vi "antonio-alexander Build.vi"(8 "error in (no error)":errorcluster) -> (0 "error out":errorcluster)   [LabVIEW 2015, in "lv-build-interface.lvlib"]
doc: "Build can be used to load a lv-builder class and build/post/deploy one or more build distributions for a loaded project."
uses:
  lv-build-interface.lvlib
  private/_controls/hmi_references.ctl
  private/_controls/hmi_states.ctl
  private/_controls/event_common.ctl
  private/_controls/event_common_command.ctl
  lv-build/public/_controls/configuration_command.ctl
  lv-builder/lv-builder.lvclass
  lv-build/lv-build.lvlib
panel:
  in  "update_version":bool
  in  "set_version":bool
  in  "select_project":bool
  in  "dependencies":bool
  in  "open_dist_folder":bool
  in  "load_class":bool
  in  "configure":bool
  in  "build":bool
  in  "post":bool
  in  "start":bool
  in  "cancel":bool
  in  "deploy":bool
  in  "exit":bool
  out "builder_class":string caption="Builder Class"
  in  "targets_artifacts_tree":string[](tree)=["0"]
  out "version":string caption="Version"
  out "git_commit_hash":string caption="Git Commit Hash"
  out "progress_bar":dbl(slide) caption="Progress" scale=0.0..100.0
  out "status":string caption="Status"
  out "project_file":string caption="Project"
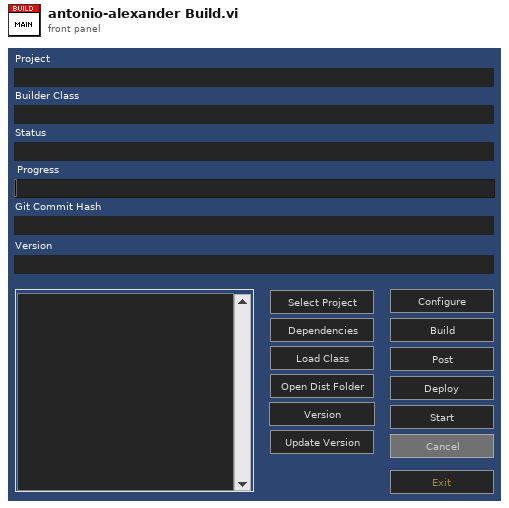
[diagram p1: front panel]
types:
  T1 = typedef "lv-build-interface.lvlib/event_common.ctl" = cluster{"command":T2, "data":variant}
  T2 = typedef "lv-build-interface.lvlib/event_common_command.ctl" = enum16{"<command>", "die", "<null>"}
  T3 = typedef "lv-build-interface.lvlib/hmi_references.ctl" = cluster{"vi_reference":refnum<vi>, "status":refnum<vi>, "progress":refnum<vi>, "tree":refnum<vi>, "project_file":refnum<vi>, "commit_hash":refnum<vi>, "version":refnum<vi>, "build":refnum<vi>, "cancel":refnum<vi>, "post":refnum<vi>, "start":refnum<vi>, "builder_class":refnum<vi>, "deploy":refnum<vi>}
  T4 = typedef "lv-build-interface.lvlib/hmi_states.ctl" = enum16{"<hmi_states>", "initialize", "check_ui", "shutdown", "<null>"}
  T5 = typedef "lv-build.lvlib/configuration_command.ctl" = enum16{"<config_command>", "read_config", "write_config", "<null>"}
  T6 = typedef "lv-build-interface.lvlib/action.ctl" = enum16{"<action>", "build", "post", "deploy", "<null>"}
  T7 = typedef "lv-build.lvlib/build_specification.ctl" = cluster{"type":T8, "build_spec_name":string, "target_name":string, "owner_name []":string[], "project_path":path, "build_destination":path, "build_artifact":path, "post_artifact":path}
  T8 = typedef "lv-build.lvlib/build_type.ctl" = enum16{"<build_type>", "application_pc", "application_rt", "installer", "llb", "lvlibp", "zip", "fpga", "<null>"}
  T9 = typedef "lv-build.lvlib/configuration.ctl" = cluster{"project_file":string, "build_class_file":string}
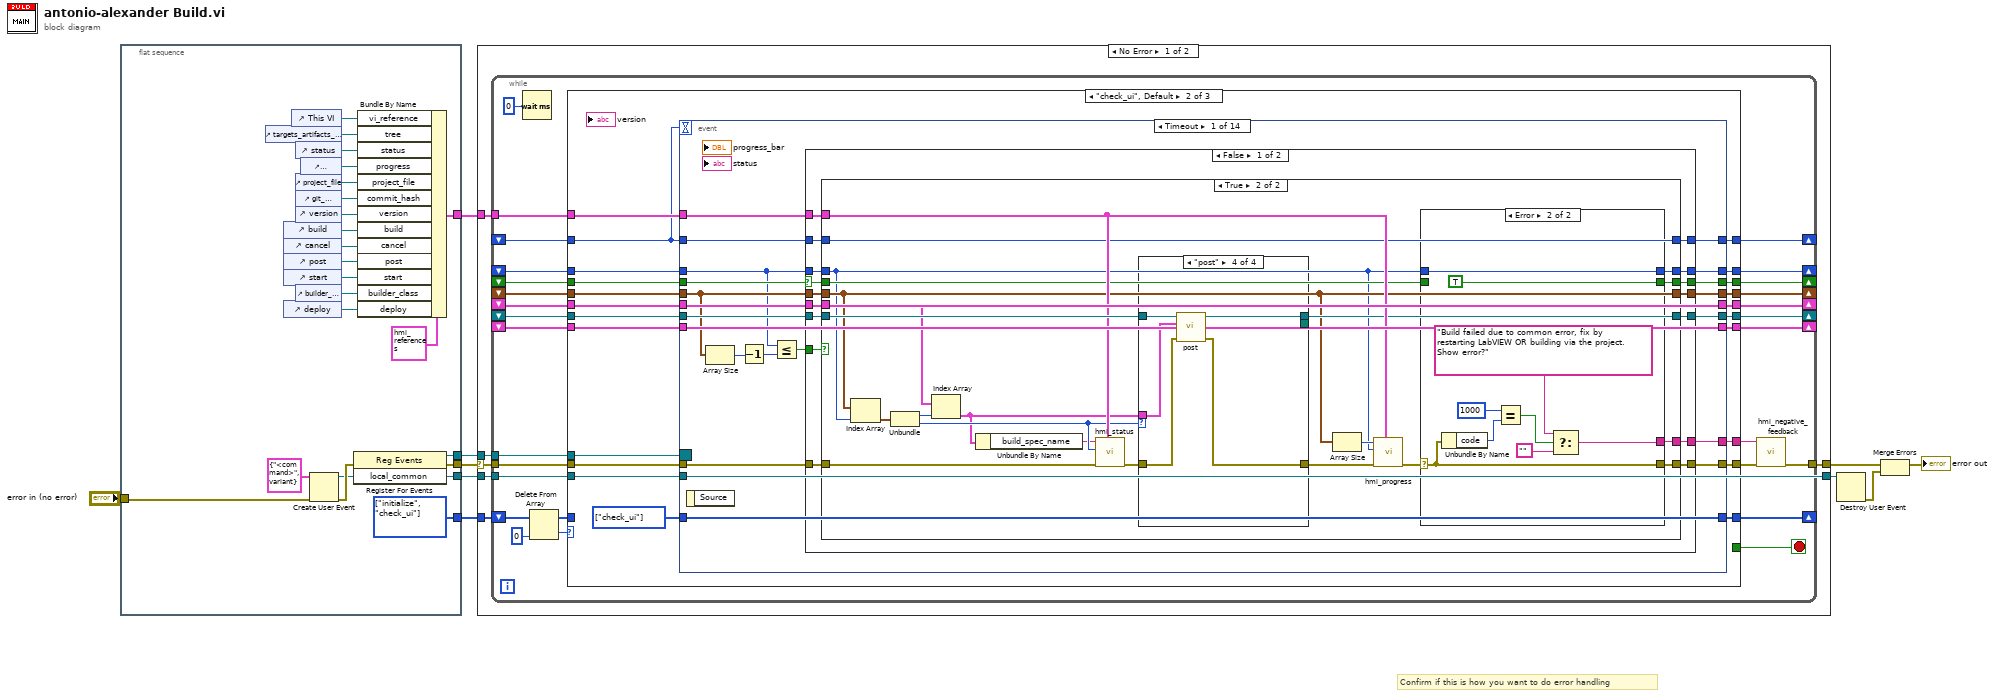
[diagram p0: block diagram]
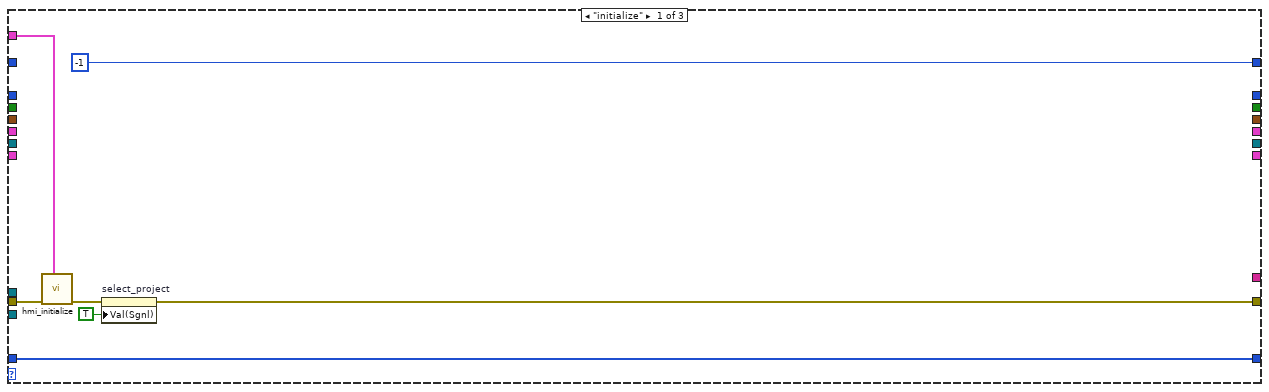
[diagram p2: hidden frame]
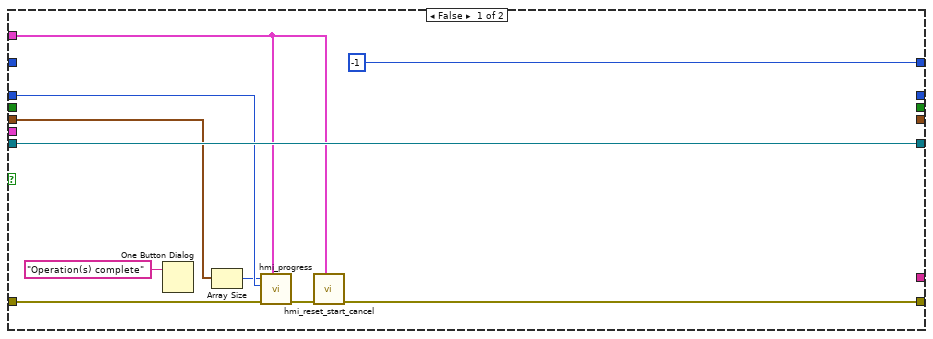
[diagram p3: hidden frame]
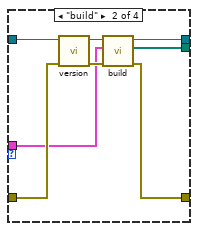
[diagram p5: hidden frame]
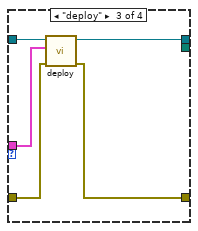
[diagram p6: hidden frame]
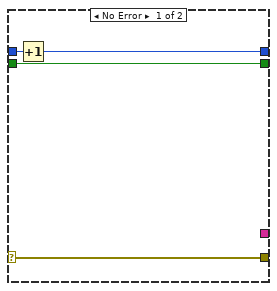
[diagram p7: hidden frame]
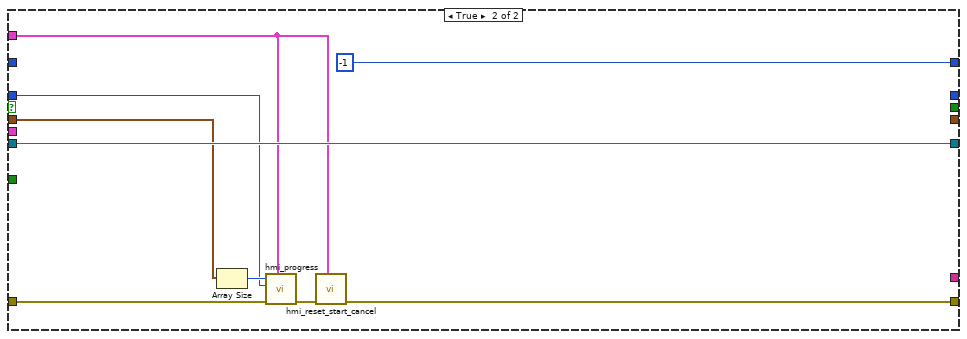
[diagram p8: hidden frame]
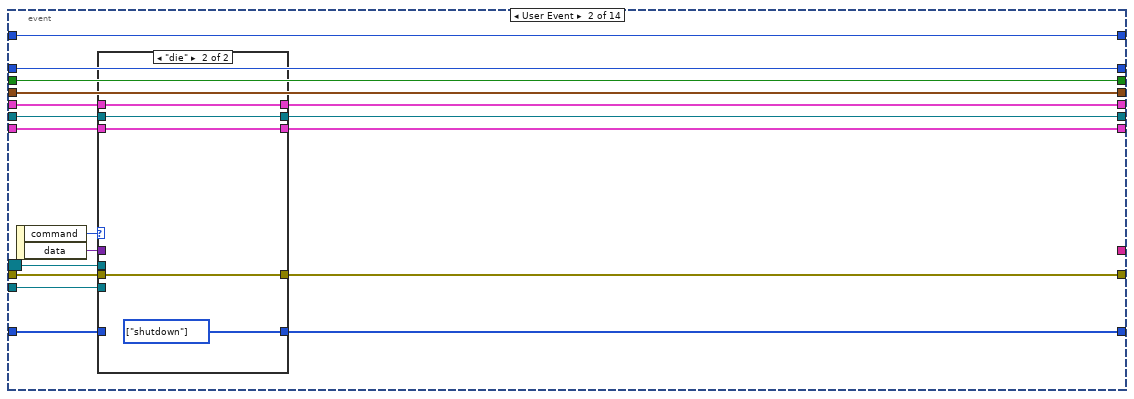
[diagram p9: hidden frame]
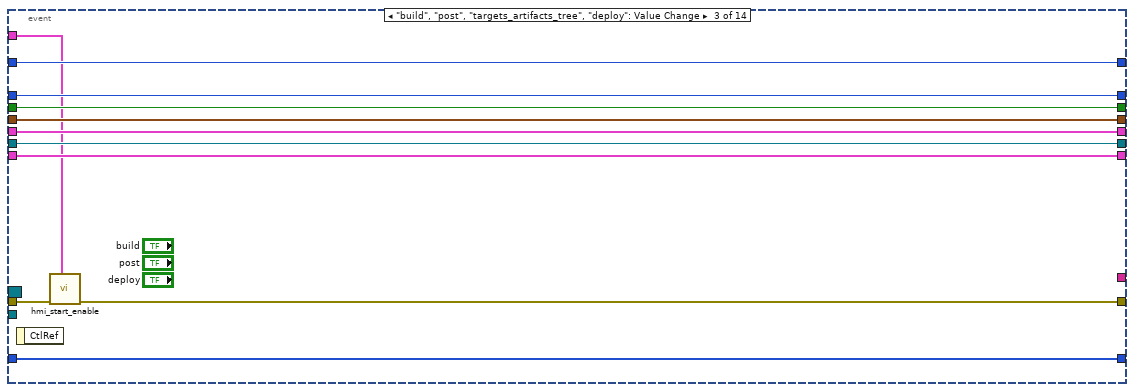
[diagram p11: hidden frame]
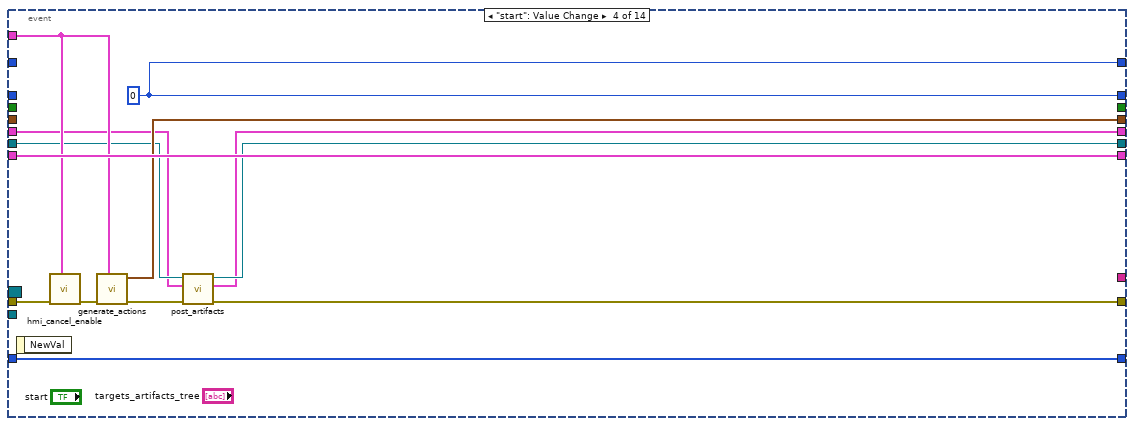
[diagram p12: hidden frame]
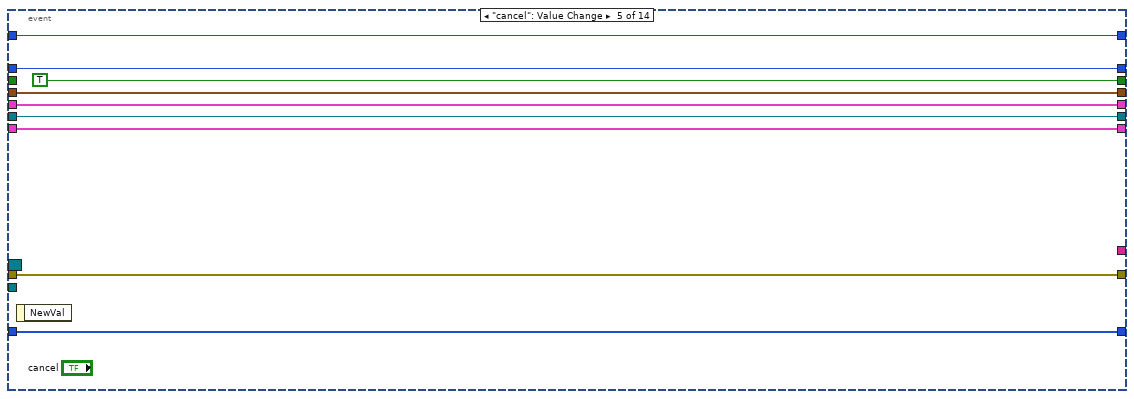
[diagram p13: hidden frame]
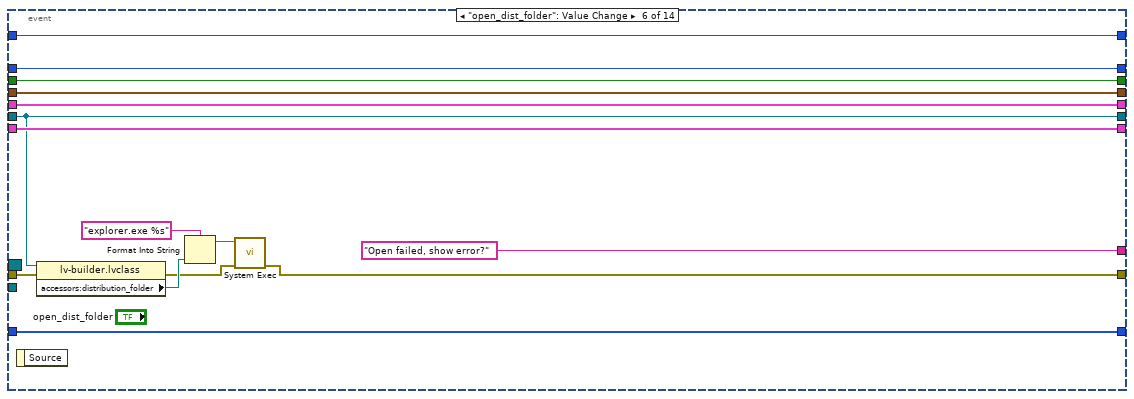
[diagram p14: hidden frame]
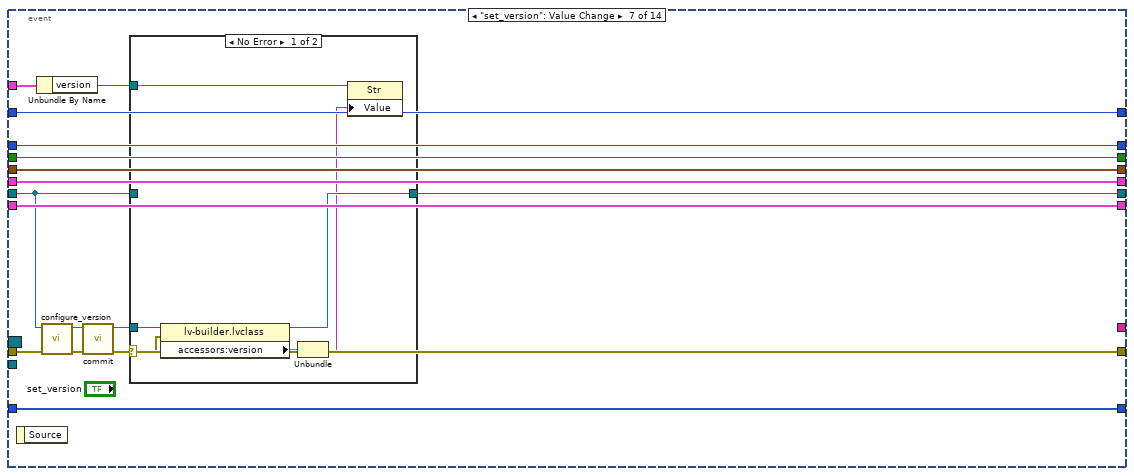
[diagram p15: hidden frame]
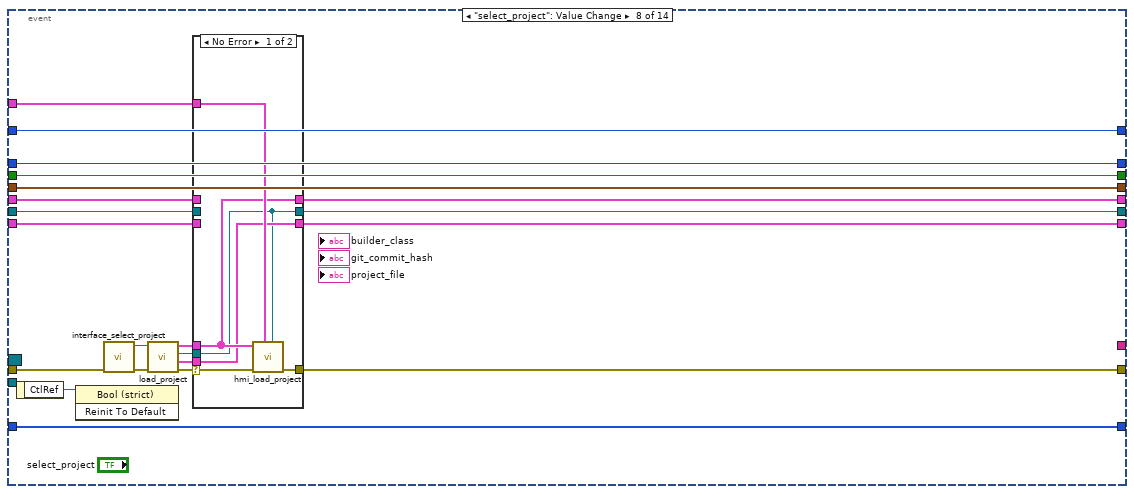
[diagram p17: hidden frame]
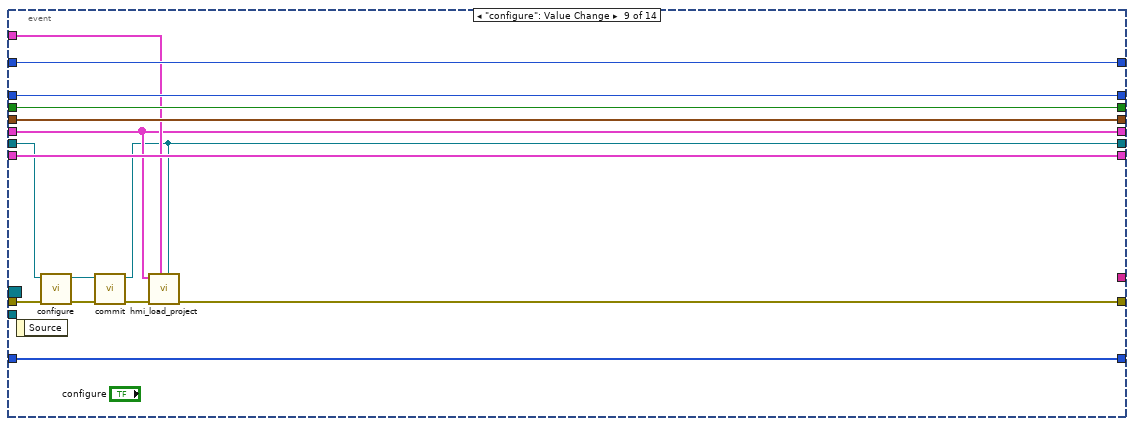
[diagram p19: hidden frame]
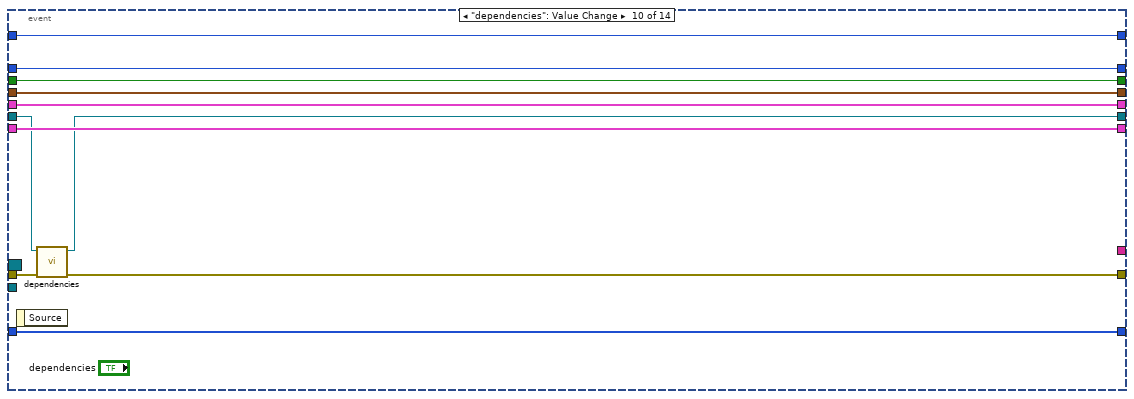
[diagram p20: hidden frame]
diagram:
  # "Confirm if this is how you want to do error handling"
  n1 = flat-sequence {
    tunnel: [w31] -> w10
    tunnel: [w29] -> w9
    tunnel: "error in (no error)" -> [w18]
    tunnel: [w17] -> w7
    tunnel: [w27] -> w6
    tunnel: [w22] -> w5
    frame #0 {
      w29 = T4[] [enum."initialize", enum."check_ui"] items=["<hmi_states>", "initialize", "check_ui", "shutdown", "<null>"]
      n2 = control-ref of="targets_artifacts_tree"() -> (w25:refnum<vi>)
      n3 = control-ref of="build"() -> (w16:refnum<vi>)
      n4 = control-ref of="cancel"() -> (w15:refnum<vi>)
      n5 = control-ref of="post"() -> (w14:refnum<vi>)
      n6 = control-ref of="start"() -> (w13:refnum<vi>)
      n7 = control-ref of="deploy"() -> (w11:refnum<vi>)
      n8 = control-ref of="This VI"() -> (w28:refnum<vi>)
      n9 = control-ref of="status"() -> (w24:refnum<vi>)
      n10 = control-ref of="project_file"() -> (w21:refnum<vi>)
      n11 = control-ref of="git_commit_hash"() -> (w20:refnum<vi>)
      n12 = control-ref of="version"() -> (w19:refnum<vi>)
      n13 = control-ref of="builder_class"() -> (w12:refnum<vi>)
      n14 = control-ref of="progress_bar"() -> (w23:refnum<vi>)
      n15 = Create User Event(user event datatype=T1 {"command"=enum."<command>", "data"=variant} ("local_common"), error in=w18) -> (user event=w22:refnum<user-event>, error out=w32:errorcluster)
      n16 = register-events(error in=w32, w22) -> (reference out=w17:refnum<event-registration>, error out=w31:errorcluster)  [unwired: 1 in]
      n17 = Bundle By Name(cluster=T3 {"vi_reference"=refnum, "status"=refnum, "progress"=refnum, "tree"=refnum, "project_file"=refnum, "commit_hash"=refnum, "version"=refnum, "build"=refnum, "cancel"=refnum, "post"=refnum, "start"=refnum, "builder_class"=refnum, "deploy"=refnum}, "vi_reference"=w28, "tree"=w25, "status"=w24, "progress"=w23, "project_file"=w21, "commit_hash"=w20, "version"=w19, "build"=w16, "cancel"=w15, "post"=w14, "start"=w13, "builder_class"=w12, "deploy"=w11) -> (w27:T3)
    }
  }
  n18 = case shown="No Error" w10 {
    selector: w10 -> [w38 w444]
    tunnel: w9 -> [w36 _]
    tunnel: [w37 w444] -> w3
    tunnel: w7 -> [w35 w442]
    tunnel: w6 -> [w34 _]
    tunnel: w5 -> [w33 w443]
    tunnel: [w33 w443] -> w4
    frame No Error {
      n19 = while {
        shift-right: [w58] -> _
        shift-left: w36 -> [w65]
        tunnel: w35 -> [w59]
        tunnel: w38 -> [w61]
        tunnel: [w48] -> w37
        tunnel: w34 -> [w57]
        tunnel: w33 -> [w56]
        shift-right: [w54] -> _
        shift-left: _ -> [w55]
        shift-right: [w52] -> _
        shift-left: _ -> [w53]
        shift-right: [w50] -> _
        shift-left: _ -> [w51]
        shift-right: [w45] -> _
        shift-left: _ -> [w47]
        shift-right: [w44] -> _
        shift-left: _ -> [w46]
        shift-right: [w42] -> _
        shift-left: _ -> [w43]
        shift-right: [w39] -> _
        shift-left: _ -> [w40]
        stop <- w60 stop-if-true
        n20 = Wait (ms)(milliseconds to wait=u32 0) -> ()  [unwired: 1 out]
        n21 = Delete From Array(array=w65, index=0) -> (deleted portion=w63:T4, array with subset deleted=w62:T4[])  [unwired: 1 in]
        n22 = case shown="\"check_ui\", Default" w63 {
          tunnel: w62 -> [w73 _ _]
          tunnel: w61 -> [w72 w95 w440]
          tunnel: [_ _ TRUE] -> w60
          tunnel: [w69 w94 w439] -> w49
          tunnel: [w73 w93 w438] -> w58
          tunnel: w59 -> [_ w91 w436]
          tunnel: w57 -> [w71 w86 w437]
          tunnel: w56 -> [_ w85 _]
          tunnel: w55 -> [_ w90 _]
          tunnel: [_ w89 _] -> w54
          tunnel: w53 -> [_ w88 _]
          tunnel: [_ w87 _] -> w52
          tunnel: w51 -> [_ w84 _]
          tunnel: [_ w83 _] -> w50
          tunnel: w47 -> [_ w82 _]
          tunnel: w46 -> [_ w81 _]
          tunnel: [_ w80 _] -> w45
          tunnel: [_ w79 _] -> w44
          tunnel: w43 -> [_ w77 w435]
          tunnel: [-1 w78 w435] -> w42
          tunnel: [_ w76 _] -> w41
          tunnel: w40 -> [_ w75 _]
          tunnel: [_ w74 _] -> w39
          frame "initialize" {
            n23 = call "hmi_initialize.vi"("hmi_references"=w71, "error in (no error)"=w72) -> ("error out"=w70:errorcluster)  [unwired: 9 in]
            n24 = property on="select_project" class="Bool (strict)"(error in=w70, "Val(Sgnl)"=TRUE ("Value (Signaling)")) -> (error out=w69:errorcluster)  [unwired: 1 in, 1 out]
          }
          frame "check_ui", Default {
            w92 = T4[] [enum."check_ui"] items=["<hmi_states>", "initialize", "check_ui", "shutdown", "<null>"]
            n25 = event shown="[0] Timeout" {
              selector: w91 -> [_ w217 _ _ _ _ _ _ _ _ _ _ _ _]
              dyn-events: _ -> [_ _ _ _ _ _ _ _ _ _ _ _ _ _]
              timeout: w77 -> [_ _ _ _ _ _ _ _ _ _ _ _ _ _]
              tunnel: w95 -> [w112 w221 w235 w253 w260 w268 w290 w324 w348 w352 w363 w400 w421 w429]
              tunnel: [w113 w218 w238 w245 w260 w272 w283 w313 w340 w351 w376 w399 w416 w428] -> w94
              tunnel: [w115 w219 w244 w257 w266 w281 w297 w325 w350 w360 w388 w409 w415 w427] -> w93
              tunnel: w92 -> [w115 w220 w244 w257 w266 w281 w297 w325 w350 w360 w388 w409 w415 w427]
              tunnel: w90 -> [w108 w216 w243 w248 w263 w280 w296 w311 w341 w361 w375 w408 w420 w434]
              tunnel: [w108 w215 w243 w247 w263 w280 w296 w310 w341 w361 w374 w408 w420 w434] -> w89
              tunnel: w88 -> [w107 w214 w242 w250 w265 w270 w282 w306 w344 w354 w373 w402 w419 w433]
              tunnel: [w105 w213 w242 w249 w265 w270 w289 w309 w338 w353 w372 w401 w419 w433] -> w87
              tunnel: w86 -> [w110 _ w234 w251 _ _ w288 w312 w342 _ w377 _ _ _]
              tunnel: w85 -> [_ w212 _ _ _ _ _ _ _ _ _ _ w417 w430]
              tunnel: w84 -> [w114 w211 w236 w256 w264 w277 w295 w307 w349 w356 w369 w407 w414 w426]
              tunnel: [w114 w210 w236 w256 w264 w277 w295 w308 w349 w356 w371 w407 w414 w426] -> w83
              tunnel: w82 -> [w111 w209 w241 _ _ w276 w294 w322 w347 w359 w387 w406 w413 w425]
              tunnel: w81 -> [w101 w208 w240 _ w262 w275 w293 w321 w346 w358 w386 w405 w412 w424]
              tunnel: [w106 w209 w241 _ TRUE w276 w294 w322 w347 w359 w387 w406 w413 w425] -> w80
              tunnel: [w109 w208 w240 w255 w262 w275 w293 w321 w346 w358 w386 w405 w412 w424] -> w79
              tunnel: w77 -> [w103 w207 w239 _ w258 w274 w292 w320 w345 w357 w385 w404 w411 w423]
              tunnel: [w102 w207 w239 w254 w258 w274 w292 w320 w345 w357 w385 w404 w411 w423] -> w78
              tunnel: [w96 _ _ _ _ "Open failed, show error?" ("dialog_text") _ _ _ _ _ _ _ _] -> w76
              tunnel: w75 -> [w99 w206 w237 _ w259 w271 w291 w305 w343 w355 w384 w403 w410 w422]
              tunnel: [w104 w206 w237 w254 w259 w271 w291 w305 w343 w355 w384 w403 w410 w422] -> w74
              event Timeout {
                n26 = event-data() -> ()  [unwired: 1 in, 1 out]
                n27 = Array Size(array=w101) -> (size(s)=w100:i32)
                n28 = Decrement(x=w100) -> (x-1=w97:i32)
                n29 = Less Or Equal?(x=w99, y=w97) -> (x <= y?=w98:bool)
                n30 = case shown="False" w111 {
                  selector: w111 -> [w129 _]
                  tunnel: [w131 w197] -> w113
                  tunnel: w112 -> [w130 w202]
                  tunnel: w110 -> [w128 w199]
                  tunnel: w101 -> [w127 w200]
                  tunnel: [w126 _] -> w109
                  tunnel: w108 -> [w125 _]
                  tunnel: w107 -> [w124 w204]
                  tunnel: [w123 _] -> w106
                  tunnel: [w122 w204] -> w105
                  tunnel: w99 -> [w121 w201]
                  tunnel: [w120 _] -> w104
                  tunnel: w103 -> [w119 _]
                  tunnel: [w118 -1] -> w102
                  tunnel: w98 -> [w117 _]
                  tunnel: [w116 _] -> w96
                  frame False {
                    n31 = case shown="True" w117 {
                      tunnel: w130 -> [w137 w162]
                      tunnel: w127 -> [w138 w147]
                      tunnel: [_ w147] -> w126
                      tunnel: [w133 w157] -> w131
                      tunnel: w124 -> [w141 w163]
                      tunnel: w128 -> [w132 w156]
                      tunnel: w129 -> [_ w155]
                      tunnel: w125 -> [_ w154]
                      tunnel: [_ w152] -> w123
                      tunnel: [w141 w150] -> w122
                      tunnel: w121 -> [w140 w146]
                      tunnel: [_ w145] -> w120
                      tunnel: w119 -> [_ w144]
                      tunnel: [-1 w144] -> w118
                      tunnel: [_ w143] -> w116
                      frame False {
                        n32 = One Button Dialog(message="Operation(s) complete" ("dialog_text")) -> ()  [unwired: 1 in, 1 out]
                        n33 = Array Size(array=w138) -> (size(s)=w135:i32)
                        n34 = call "hmi_progress.vi"("hmi_references"=w132, "error in (no error)"=w137, "current_index"=w140, "total_operations"=w135) -> ("error out"=w134:errorcluster)  [unwired: 7 in]
                        n35 = call "hmi_reset_start_cancel.vi"("hmi_references"=w132, "error in (no error)"=w134) -> ("error out"=w133:errorcluster)  [unwired: 9 in]
                      }
                      frame True {
                        n36 = Index Array(array=w147, index=w146) -> (element=w153:cluster{"index":i32, "action":T6})
                        n37 = Unbundle(w153) -> ("index"=w151:i32, "action"=w149:T6)
                        n38 = Index Array(array=w154, index=w151) -> (element=w142:T7)
                        n39 = Unbundle By Name(w142) -> ("build_spec_name"=w148:string)
                        n40 = call "hmi_status.vi"("hmi_references"=w156, "error in (no error)"=w162, "action"=w149, "build_spec.build_spec_name"=w148) -> ("error out"=w161:errorcluster)  [unwired: 7 in]
                        n41 = case shown="\"post\"" w149 {
                          tunnel: w161 -> [w165 w173 w178 w183]
                          tunnel: [w165 w171 w177 w182] -> w160
                          tunnel: w163 -> [w164 w168 w175 w179]
                          tunnel: w142 -> [_ w166 w176 w181]
                          tunnel: [w164 w170 w174 w180] -> w150
                          tunnel: [_ w169 _ _] -> _
                          frame Default {
                          }
                          frame "build" {
                            n42 = call-dynamic "version.vi"("error in (no error)"=w173, "lv-builder in"=w168) -> ("error out"=w172:errorcluster, "lv-builder out"=w167:refnum<class "lv-builder.lvclass">)  [unwired: 8 in]
                            n43 = call-dynamic "build.vi"("error in (no error)"=w172, "build_spec"=w166, "lv-build-default in"=w167) -> ("error out"=w171:errorcluster, "[] generated_files"=w169:path[], "lv-build-default out"=w170:refnum<class "lv-builder.lvclass">)  [unwired: 6 in]
                          }
                          frame "deploy" {
                            n44 = call-dynamic "deploy.vi"("error in (no error)"=w178, "build_spec"=w176, "lv-builder in"=w175) -> ("error out"=w177:errorcluster, "lv-builder out"=w174:refnum<class "lv-builder.lvclass">)  [unwired: 7 in]
                          }
                          frame "post" {
                            n45 = call-dynamic "post.vi"("error in (no error)"=w183, "build_spec"=w181, "lv-build-default in"=w179) -> ("error out"=w182:errorcluster, "lv-build-default out"=w180:refnum<class "lv-builder.lvclass">)  [unwired: 7 in]
                          }
                        }
                        n46 = Array Size(array=w147) -> (size(s)=w159:i32)
                        n47 = call "hmi_progress.vi"("hmi_references"=w156, "error in (no error)"=w160, "current_index"=w146, "total_operations"=w159) -> ("error out"=w158:errorcluster)  [unwired: 7 in]
                        n48 = case shown="Error" w158 {
                          selector: w158 -> [w187 w194]
                          tunnel: [w187 w194] -> w157
                          tunnel: w155 -> [w186 _]
                          tunnel: [w186 TRUE] -> w152
                          tunnel: w146 -> [w185 w195]
                          tunnel: [w184 w195] -> w145
                          tunnel: [_ w188] -> w143
                          frame No Error {
                            n49 = Increment(x=w185) -> (x+1=w184:i32)
                          }
                          frame Error {
                            n50 = Unbundle By Name(w194) -> ("code"=w193:i32)
                            n51 = Equal?(x=1000, y=w193) -> (x = y?=w191:bool)
                            n52 = Select(t="Build failed due to common error, fix by restarting LabVIEW OR building via the project.  Show error?", s=w191, f="") -> (s? t:f=w188:string)
                          }
                        }
                      }
                    }
                  }
                  frame True {
                    n53 = Array Size(array=w200) -> (size(s)=w203:i32)
                    n54 = call "hmi_progress.vi"("hmi_references"=w199, "error in (no error)"=w202, "current_index"=w201, "total_operations"=w203) -> ("error out"=w198:errorcluster)  [unwired: 7 in]
                    n55 = call "hmi_reset_start_cancel.vi"("hmi_references"=w199, "error in (no error)"=w198) -> ("error out"=w197:errorcluster)  [unwired: 9 in]
                  }
                }
              }
              event User Event {
                n56 = event-data() -> ("command"=w223:T2, "data"=w222:variant)  [unwired: 1 in]
                n57 = case shown="\"die\"" w223 {
                  tunnel: [w228 w233] -> w219
                  tunnel: w220 -> [w228 _]
                  tunnel: w221 -> [w227 w232]
                  tunnel: [w227 w232] -> w218
                  tunnel: w222 -> [_ _]
                  tunnel: w217 -> [_ _]
                  tunnel: w216 -> [w226 w231]
                  tunnel: [w226 w231] -> w215
                  tunnel: w214 -> [w225 w230]
                  tunnel: [w225 w230] -> w213
                  tunnel: w212 -> [_ _]
                  tunnel: w211 -> [w224 w229]
                  tunnel: [w224 w229] -> w210
                  frame Default {
                  }
                  frame "die" {
                    w233 = T4[] [enum."shutdown"] items=["<hmi_states>", "initialize", "check_ui", "shutdown", "<null>"]
                  }
                }
              }
              event "build", "post", "targets_artifacts_tree", "deploy": Value Change {
                n58 = event-data() -> ()  [unwired: 1 in, 1 out]
                n59 = call "hmi_start_enable.vi"("hmi_references"=w234, "error in (no error)"=w235) -> ("error out"=w238:errorcluster)  [unwired: 9 in]
              }
              event "start": Value Change {
                w254 = 0
                n60 = event-data() -> ()  [unwired: 1 in, 1 out]
                n61 = call "hmi_cancel_enable.vi"("hmi_references"=w251, "error in (no error)"=w253) -> ("error out"=w252:errorcluster)  [unwired: 9 in]
                n62 = call "generate_actions.vi"("hmi_references"=w251, "error in (no error)"=w252) -> ("error out"=w246:errorcluster, "actions []"=w255:cluster{"index":i32, "action":T6}[])  [unwired: 8 in]
                n63 = call-dynamic "post_artifacts.vi"("error in (no error)"=w246, "build_spec_info [] in"=w248, "lv-builder in"=w250) -> ("error out"=w245:errorcluster, "build_spec_info [] out"=w247:T7[], "lv-builder out"=w249:refnum<class "lv-builder.lvclass">)  [unwired: 6 in]
              }
              event "cancel": Value Change {
                n64 = event-data() -> ()  [unwired: 1 in, 1 out]
              }
              event "open_dist_folder": Value Change {
                n65 = event-data() -> ()  [unwired: 1 in, 1 out]
                n66 = property class="lv-builder.lvclass"(reference=w270, error in=w268) -> (error out=w267:errorcluster, "accessors:distribution_folder"=w269:path)  [unwired: 1 out]
                n67 = Format Into String(format string="explorer.exe %s", w269) -> (resulting string=w279:string)  [unwired: 2 in, 1 out]
                n68 = call <vilib>:"System Exec.vi"("error in (no error)"=w267, "command line"=w279) -> ("error out"=w272:errorcluster)  [unwired: 6 in, 3 out]
              }
              event "set_version": Value Change {
                n69 = event-data() -> ()  [unwired: 1 in, 1 out]
                n70 = Unbundle By Name(w288) -> ("version"=w287:refnum<vi>)
                n71 = call-dynamic "configure_version.vi"("error in (no error)"=w290, "lv-build-default in"=w282) -> ("error out"=w285:errorcluster, "lv-build-default out"=w286:refnum<class "lv-builder.lvclass">)  [unwired: 8 in]
                n72 = call-dynamic "commit.vi"("error in (no error)"=w285, "lv-builder in"=w286) -> ("error out"=w283:errorcluster, "lv-builder out"=w284:refnum<class "lv-builder.lvclass">)  [unwired: 8 in]
                n73 = case shown="No Error" w283 {
                  selector: w283 -> [w299 _]
                  tunnel: [w302 w304] -> w289
                  tunnel: w287 -> [w301 _]
                  tunnel: w284 -> [w298 _]
                  tunnel: w282 -> [_ w304]
                  frame No Error {
                    n74 = property class="lv-builder.lvclass"(reference=w298, error in=w299) -> (reference out=w302:refnum<class "lv-builder.lvclass">, "accessors:version"=w303:cluster{"data":variant, "string":string})  [unwired: 1 out]
                    n75 = Unbundle(w303) -> ("string"=w300:string)  [unwired: 1 out]
                    n76 = property class="Str"(reference=w301, "Value"=w300) -> ()  [unwired: 1 in, 2 out]
                  }
                  frame Error {
                  }
                }
              }
              event "select_project": Value Change {
                n77 = event-data() -> ("CtlRef"=w323:refnum<vi>)  [unwired: 1 in]
                n78 = invoke on="Invoke Node" class="Bool (strict)" method="Reinit To Default"(reference=w323) -> ()  [unwired: 2 in, 3 out]
                n79 = call "interface_select_project.vi"("error in (no error)"=w324) -> ("error out"=w319:errorcluster, "project_path"=w318:path)  [unwired: 9 in]
                n80 = call "load_project.vi"("error in (no error)"=w319, "project_file"=w318) -> ("error out"=w314:errorcluster, "config"=w315:T9, "lv-builder out"=w316:refnum<class "lv-builder.lvclass">, "build_spec_info []"=w317:T7[])  [unwired: 6 in]
                n81 = case shown="No Error" w314 {
                  selector: w314 -> [w331 w334]
                  tunnel: [w330 w334] -> w313
                  tunnel: w311 -> [_ w335]
                  tunnel: [w328 w335] -> w310
                  tunnel: [w327 w333] -> w308
                  tunnel: w312 -> [w329 _]
                  tunnel: w316 -> [w326 _]
                  tunnel: w315 -> [w327 _]
                  tunnel: w317 -> [w328 _]
                  tunnel: [w326 w332] -> w309
                  tunnel: w307 -> [_ w333]
                  tunnel: w306 -> [_ w332]
                  frame No Error {
                    n82 = call "hmi_load_project.vi"("lv-builder.lvlib:lv-builder.lvclass"=w326, "hmi_references"=w329, "error in (no error)"=w331, "build_spec []"=w328) -> ("error out"=w330:errorcluster)  [unwired: 7 in]
                  }
                  frame Error {
                  }
                }
              }
              event "configure": Value Change {
                n83 = event-data() -> ()  [unwired: 1 in, 1 out]
                n84 = call-dynamic "configure.vi"("error in (no error)"=w348, "lv-build-default in"=w344) -> ("error out"=w337:errorcluster, "lv-build-default out"=w339:refnum<class "lv-builder.lvclass">)  [unwired: 8 in]
                n85 = call-dynamic "commit.vi"("error in (no error)"=w337, "lv-builder in"=w339) -> ("error out"=w336:errorcluster, "lv-builder out"=w338:refnum<class "lv-builder.lvclass">)  [unwired: 8 in]
                n86 = call "hmi_load_project.vi"("lv-builder.lvlib:lv-builder.lvclass"=w338, "hmi_references"=w342, "error in (no error)"=w336, "build_spec []"=w341) -> ("error out"=w340:errorcluster)  [unwired: 7 in]
              }
              event "dependencies": Value Change {
                n87 = event-data() -> ()  [unwired: 1 in, 1 out]
                n88 = call-dynamic "dependencies.vi"("error in (no error)"=w352, "lv-builder in"=w354) -> ("error out"=w351:errorcluster, "lv-builder out"=w353:refnum<class "lv-builder.lvclass">)  [unwired: 8 in]
              }
              event "load_class": Value Change {
                n89 = event-data() -> ()  [unwired: 1 in, 1 out]
                n90 = call "interface_select_class.vi"("error in (no error)"=w363) -> ("error out"=w362:errorcluster, "builder_class file"=w364:path)  [unwired: 9 in]
                n91 = Path To String(path=w364) -> (string=w368:string)
                n92 = Bundle By Name(cluster=w369, "build_class_file"=w368) -> (w367:T9)
                n93 = call "configuration.vi"("command"=configuration_command."write_config", "error in (no error)"=w362, "config in"=w367) -> ("error out"=w365:errorcluster, "config out"=w366:T9)  [unwired: 7 in]
                n94 = Unbundle By Name(w366) -> ("project_file"=w383:string)
                n95 = String To Path(string=w383) -> (path=w382:path)
                n96 = call "load_project.vi"("error in (no error)"=w365, "project_file"=w382) -> ("error out"=w381:errorcluster, "config"=w380:T9, "lv-builder out"=w379:refnum<class "lv-builder.lvclass">, "build_spec_info []"=w378:T7[])  [unwired: 6 in]
                n97 = case shown="No Error" w381 {
                  selector: w381 -> [w394 w398]
                  tunnel: [w390 w398] -> w376
                  tunnel: [w392 w397] -> w374
                  tunnel: [w389 w395] -> w371
                  tunnel: w377 -> [w393 _]
                  tunnel: w379 -> [w391 _]
                  tunnel: w380 -> [w389 _]
                  tunnel: w378 -> [w392 _]
                  tunnel: [w391 w396] -> w372
                  tunnel: w375 -> [_ w397]
                  tunnel: w373 -> [_ w396]
                  tunnel: w369 -> [_ w395]
                  frame No Error {
                    n98 = call "hmi_load_project.vi"("lv-builder.lvlib:lv-builder.lvclass"=w391, "hmi_references"=w393, "error in (no error)"=w394, "build_spec []"=w392) -> ("error out"=w390:errorcluster)  [unwired: 7 in]
                  }
                  frame Error {
                  }
                }
              }
              event "update_version": Value Change {
                n99 = event-data() -> ()  [unwired: 1 in, 2 out]
                n100 = call-dynamic "version.vi"("error in (no error)"=w400, "lv-builder in"=w402) -> ("error out"=w399:errorcluster, "lv-builder out"=w401:refnum<class "lv-builder.lvclass">)  [unwired: 8 in]
              }
              event "exit": Value Change {
                n101 = event-data() -> ()  [unwired: 1 in, 1 out]
                n102 = Generate User Event(user event=w417, event data cluster=T1 {"command"=enum."die", "data"=variant} ("event data"), error in=w421) -> (error out=w416:errorcluster)  [unwired: 1 in, 1 out]
              }
              event Panel Close? {
                n103 = event-data() -> ()  [unwired: 1 in, 1 out]
                n104 = Generate User Event(user event=w430, event data cluster=T1 {"command"=enum."die", "data"=variant} ("event data"), error in=w429) -> (error out=w428:errorcluster)  [unwired: 1 in, 1 out]
                n105 = event-data("Discard?"=TRUE) -> ()  [unwired: 1 in, 1 out]
              }
            }
          }
          frame "shutdown" {
            w438 = T4[] [enum."shutdown"] items=["<hmi_states>", "initialize", "check_ui", "shutdown", "<null>"]
            n106 = Unregister For Events(event registration refnum=w436) -> ()  [unwired: 1 in, 1 out]
            n107 = call "hmi_shutdown.vi"("hmi_references"=w437, "error in (no error)"=w440) -> ("error out"=w439:errorcluster)  [unwired: 9 in]
          }
        }
        n108 = call "hmi_negative_feedback.vi"("error in (no error)"=w49, "dialog_text"=w41) -> ("error out"=w48:errorcluster)  [unwired: 9 in]
      }
    }
    frame Error {
      n109 = Unregister For Events(event registration refnum=w442) -> ()  [unwired: 1 in, 1 out]
    }
  }
  n110 = Destroy User Event(user event=w4) -> (error out=w2:errorcluster)  [unwired: 1 in]
  n111 = Merge Errors(w3, w2) -> (→"error out":errorcluster)
